vi "Facade 4.vi"(0 "Data In":T11, 2 "Display State In":T2, 3 "Container State":T10) -> (6 "Data Out":T11, 7 "Display State Out":T2, 8 "Action":T1)   [LabVIEW 2011, in "Action select.xctl"]
uses:
  Action select.xctl
  Data 4.ctl
  <vilib>/_xctls/Container State.ctl
  State 4.ctl
  Action colleciton cluster.ctl
  Action common elements.ctl
  Action adjuster type.ctl
  Action type.ctl
  General command list.ctl
  PCP interface/High Level/PCP High Level Commands.ctl
  Tool/Stroker/def/Tool specific commands.ctl
  <vilib>/_xctls/Action.ctl
  <vilib>/_xctls/XControlSupport.lvlib
panel:
  in  "Value":dbl
  in  "Action":u16(ring)
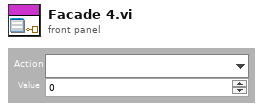
[diagram p1: front panel]
types:
  T1 = typedef "XControlSupport.lvlib/Action.ctl" = cluster{"Data Changed?":bool, "State Changed?":bool, "Action Name":string}
  T2 = typedef "Action select.xctl/State 4.ctl" = cluster{"Actions":T3[]}
  T3 = typedef "Action colleciton cluster.ctl" = cluster{"common":T4, "Action type":T6, "General command":T7, "PCP command":T8, "Tool command":T9}
  T4 = typedef "Action common elements.ctl" = cluster{"Name":string, "Adjuster type":T5, "Adjuster double default value":dbl}
  T5 = typedef "Action adjuster type.ctl" = enum16{"Non", "Double"}
  T6 = typedef "Action type.ctl" = enum16{"General", "PCP command", "Tool command"}
  T7 = typedef "General command list.ctl" = enum16{"No action"}
  T8 = typedef "PCP High Level Commands.ctl" = enum16{"HVPSU HV ON", "HVPSU HV OFF", "PCP PC", "PCP Local", "Update Motor Voltage", "Update Cable Resistance", "Final Motor Voltage", "Final Resistance"}
  T9 = typedef "Tool specific commands.ctl" = enum16{"controller relay 1 on", "controller relay 1 off", "controller relay 2 on", "controller relay 2 off", "Solonoid 1 (master) on", "Solonoid 1 (master) off", "Solonoid 2 (Stroker) on", "Solonoid 2 (Stroker) off", "Solonoid 3 (Anchor) on", "Solonoid 3 (Anchor) off", "Controller relay 1 & 2 on", "Controller relay 1 & 2 off", "Controller relay 1 on, 2 off", "Controller relay 1 off, 2 on", "STROKER tool: Stop Force Mon", "High-G Stop", "High-G Get data", "High-G Stop Get data", "STROKER tool: Stroke out", "STROKER tool: Stroke in", "STROKER tool: Stroke stop", "STROKER tool: Stroke go to", "STROKER tool: Stop Homing", "STROKER tool: Start Force Mon dir in", "STROKER tool: Start Force Mon dir out", "Controller STOP"}
  T10 = typedef "XControlSupport.lvlib/Container State.ctl" = cluster{"Indicator?":bool, "Run Mode?":bool, " Refnum":refnum<vi>}
  T11 = typedef "Action select.xctl/Data 4.ctl" = cluster{"Action index":i32, "Data":dbl}
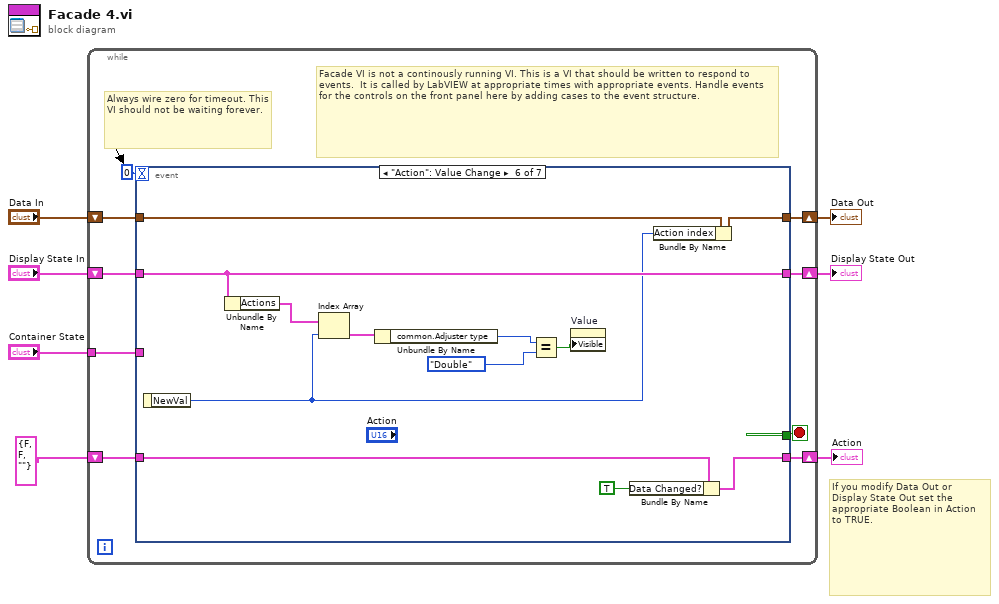
[diagram p0: block diagram]
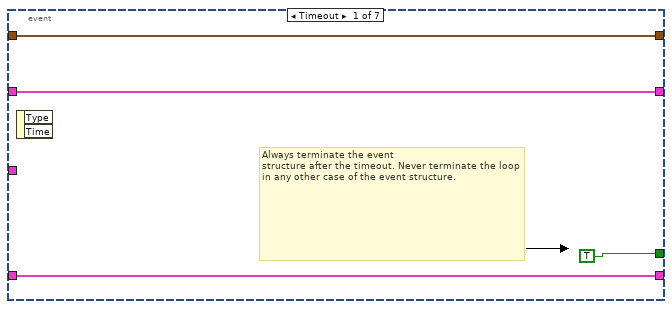
[diagram p2: hidden frame]
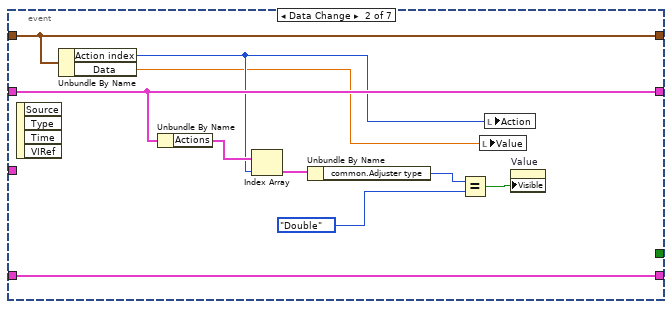
[diagram p3: hidden frame]
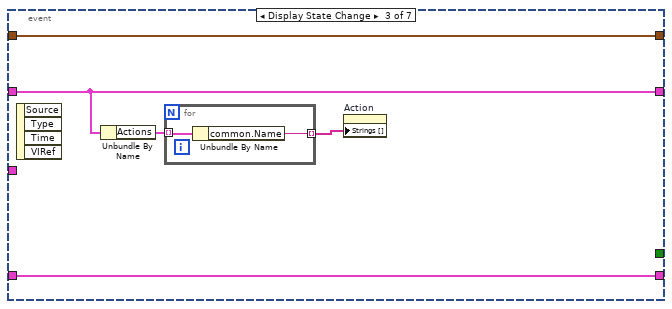
[diagram p4: hidden frame]
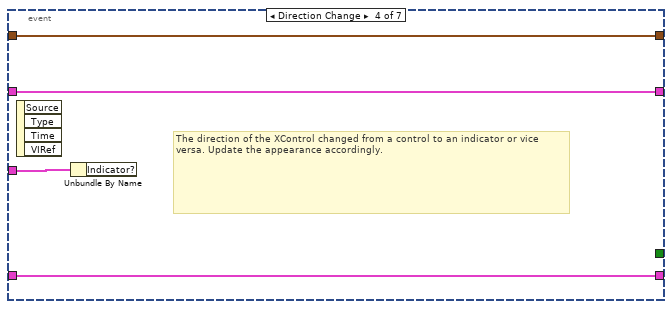
[diagram p5: hidden frame]
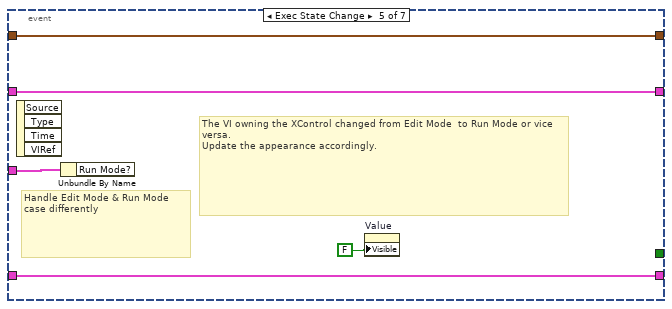
[diagram p6: hidden frame]
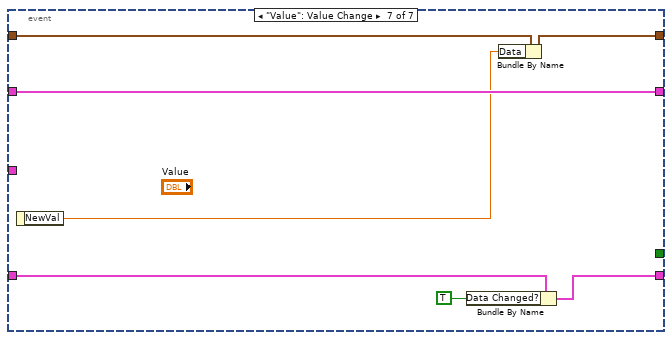
[diagram p7: hidden frame]
diagram:
  # "If you modify Data Out or\nDisplay State Out set the\nappropriate Boolean in Action\nto TRUE."
  n1 = while {
    shift-right: [w15] -> w4
    shift-left: "Display State In" -> [w16]
    tunnel: "Container State" -> [w12]
    shift-right: [w10] -> w7
    shift-left: "Data In" -> [w11]
    shift-right: [w8] -> w2
    shift-left: T1 {"Data Changed?"=FALSE, "State Changed?"=FALSE, "Action Name"=""} ("Action") -> [w9]
    stop <- w14 stop-if-true
    # "Facade VI is not a continously running VI. This is a VI that should be written to respond to events.  It is called by LabVIEW at appropriate times with appropriate events. Handle events for the controls on the front panel here by adding cases to the event structure."
    # "Always wire zero for timeout. This\nVI should not be waiting forever."
    n2 = event shown="[5] \"Action\": Value Change" {
      selector: _ -> [_ _ _ _ _ _ _]
      dyn-events: _ -> [_ _ _ _ _ _ _]
      timeout: 0 -> [_ _ _ _ _ _ _]
      tunnel: w16 -> [w18 w25 w33 w40 w45 w56 w64]
      tunnel: [w18 w25 w33 w40 w45 w56 w64] -> w15
      tunnel: [TRUE _ _ _ _ _ _] -> w14
      tunnel: w12 -> [_ _ _ w41 w46 _ _]
      tunnel: w11 -> [w17 w24 w35 w39 w44 w58 w65]
      tunnel: [w17 w24 w35 w39 w44 w57 w60] -> w10
      tunnel: [w19 w30 w34 w38 w43 w47 w62] -> w8
      tunnel: w9 -> [w19 w30 w34 w38 w43 w48 w63]
      event Timeout {
        # "Always terminate the event\nstructure after the timeout. Never terminate the loop in any other case of the event structure."
        n3 = event-data() -> ()  [unwired: 1 in, 2 out]
      }
      event Data Change {
        n4 = event-data() -> ()  [unwired: 1 in, 4 out]
        n5 = Unbundle By Name(w24) -> ("Action index"=w23:i32, "Data"=w22:dbl)
        n6 = Unbundle By Name(w25) -> ("Actions"=w29:T3[])
        n7 = Index Array(array=w29, index=w23) -> (element=w28:T3)
        n8 = Unbundle By Name(w28) -> ("common.Adjuster type"=w27:T5)
        n9 = Equal?(x=w27, y=Action_adjuster_type."Double") -> (x = y?=w21:bool)
        n10 = local write "Value"(w22) -> ()
        n11 = local write "Action"(w23) -> ()
        n12 = property on="Value" class="DigNum (strict)"("Visible"=w21) -> ()  [unwired: 2 in, 2 out]
      }
      event Display State Change {
        n13 = event-data() -> ()  [unwired: 1 in, 4 out]
        n14 = Unbundle By Name(w33) -> ("Actions"=w32:T3[])
        n15 = for {
          tunnel: w32 -> [w37] mode=indexing
          tunnel: [w36] -> w31 mode=indexing
          n16 = Unbundle By Name(w37) -> ("common.Name"=w36:string)
        }
        n17 = property on="Action" class="Ring (strict)"("Strings []"=w31) -> ()  [unwired: 2 in, 2 out]
      }
      event Direction Change {
        # "The direction of the XControl changed from a control to an indicator or vice versa. Update the appearance accordingly."
        n18 = event-data() -> ()  [unwired: 1 in, 4 out]
        n19 = Unbundle By Name(w41) -> ()  [unwired: 1 out]
      }
      event Exec State Change {
        # "The VI owning the XControl changed from Edit Mode  to Run Mode or vice versa.\nUpdate the appearance accordingly."
        # "Handle Edit Mode & Run Mode\ncase differently"
        n20 = event-data() -> ()  [unwired: 1 in, 4 out]
        n21 = Unbundle By Name(w46) -> ()  [unwired: 1 out]
        n22 = property on="Value" class="DigNum (strict)"("Visible"=FALSE) -> ()  [unwired: 2 in, 2 out]
      }
      event "Action": Value Change {
        n23 = event-data() -> ("NewVal"=w54:u16)  [unwired: 1 in]
        n24 = Unbundle By Name(w56) -> ("Actions"=w55:T3[])
        n25 = Index Array(array=w55, index=w54) -> (element=w53:T3)
        n26 = Unbundle By Name(w53) -> ("common.Adjuster type"=w52:T5)
        n27 = Equal?(x=w52, y=Action_adjuster_type."Double") -> (x = y?=w50:bool)
        n28 = property on="Value" class="DigNum (strict)"("Visible"=w50) -> ()  [unwired: 2 in, 2 out]
        n29 = Bundle By Name(cluster=w48, "Data Changed?"=TRUE) -> (w47:T1)
        n30 = Bundle By Name(cluster=w58, "Action index"=w54) -> (w57:T11)
      }
      event "Value": Value Change {
        n31 = event-data() -> ("NewVal"=w59:dbl)  [unwired: 1 in]
        n32 = Bundle By Name(cluster=w63, "Data Changed?"=TRUE) -> (w62:T1)
        n33 = Bundle By Name(cluster=w65, "Data"=w59) -> (w60:T11)
      }
    }
  }
  "Display State Out" <- w4
  "Data Out" <- w7
  "Action" <- w2
